vi "Write Set PCC Transition Msg.vi"(10 "Set PCC Transition Msg":refnum<class "Set PCC Transition Msg.lvclass">, 11 "SCADA Sub Abstract in":refnum<class "Device Communication and Control Abstract.lvclass">) -> (3 "SCADA Sub Abstract out":refnum<class "Device Communication and Control Abstract.lvclass">)   [LabVIEW 2018, in "Device Communication and Control Abstract Actor.lvlib" / "Device Communication and Control Abstract.lvclass"]
uses:
  Device Communication and Control Abstract.lvclass
  Device Communication and Control Abstract Messages/Set PCC Transition Msg/Set PCC Transition Msg.lvclass
  Device Communication and Control Abstract.lvclass/Device Communication and Control Abstract.ctl
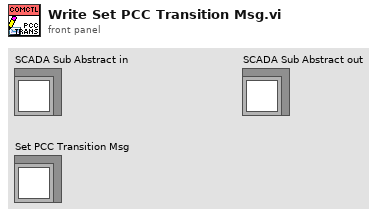
[diagram p1: front panel]
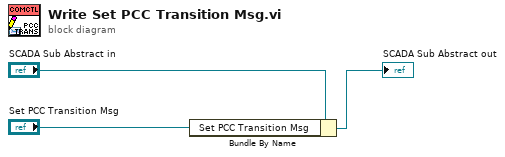
[diagram p0: block diagram]
diagram:
  n1 = Bundle By Name(cluster="SCADA Sub Abstract in", "Set PCC Transition Msg"="Set PCC Transition Msg") -> (→"SCADA Sub Abstract out":refnum<class "Device Communication and Control Abstract.lvclass">)
